vi "ChangeTblBgColor.vi"(9 "reference":refnum<vi>, 10 "Row":i32, 11 "input string":string) -> ()   [LabVIEW 2010]
uses:
  <vilib>/Utility/miscctls.llb/LVRowAndColumnTypeDef.ctl
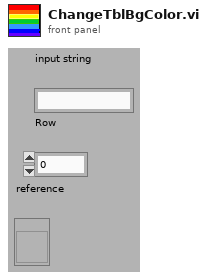
[diagram p1: front panel]
types:
  T1 = typedef "LVRowAndColumnTypeDef.ctl" = cluster{"Row":i32, "Column":i32}
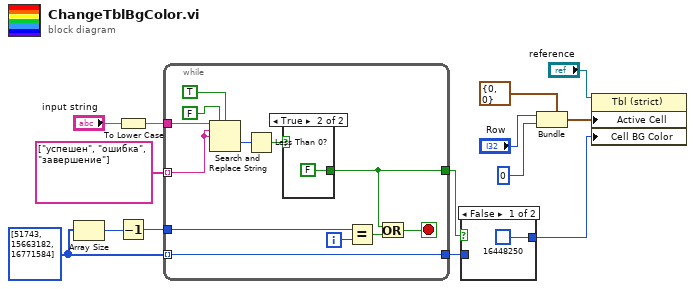
[diagram p0: block diagram]
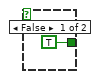
[diagram p3: hidden frame]
diagram:
  w11 = u32[] [51743, 15663182, 16771584]
  n1 = Array Size(array=w11) -> (size(s)=w7:i32)
  n2 = To Lower Case(string="input string") -> (all lower case string=w12:string)
  n3 = Decrement(x=w7) -> (x-1=w6:i32)
  n4 = while {
    tunnel: string[] ["успешен", "ошибка", "завершение"] -> [w23] mode=indexing
    tunnel: w12 -> [w22]
    tunnel: w11 -> [w15] mode=indexing
    tunnel: w6 -> [w20]
    tunnel: [w16] -> w5
    tunnel: [w15] -> w4
    i -> [w17]
    stop <- w18 stop-if-true
    n5 = Search and Replace String(replace all?=FALSE ("replace all? (F)"), case sensitive?=TRUE ("ignore case? (F)"), input string=w22, search string=w23, replace string=w23) -> (offset past replacement=w24:i32)  [unwired: 3 in, 3 out]
    n6 = Less Than 0?(x=w24) -> (x < 0?=w21:bool)
    n7 = case shown="True" w21 {
      tunnel: [TRUE FALSE] -> w16
      frame False {
      }
      frame True {
      }
    }
    n8 = Equal?(x=w20, y=w17) -> (x = y?=w19:bool)
    n9 = Or(x=w16, y=w19) -> (x .or. y?=w18:bool)
  }
  n10 = case shown="False" w5 {
    tunnel: w4 -> [_ w30]
    tunnel: [u32 16448250 ("Success") w30] -> w1
    frame False {
    }
    frame True {
    }
  }
  n11 = Bundle(cluster=T1 {"Row"=0, "Column"=0} ("Active Cell:Active Cell"), "Row"="Row", "Column"=0) -> (w2:T1)
  n12 = property class="Tbl (strict)"(reference="reference", "Active Cell"=w2, "Cell BG Color"=w1) -> ()  [unwired: 1 in, 2 out]
